vi "Add Transfer Group with Children v2.vi"(6 "Plugin Decimation (1)":u64=1, 7 "Transfer Group configuration":T1={"name"="", "direction"=enum."Tx", "cycle timing"={"priority"=0, "decimation"=1, "offset"=0}, "thread index"=-1, "settings"=[], "Transfers"=[], "timeout behavior"=enum."Increment Late Count"} {"Transfers"."channels"."string offset" format="%d bytes"}, 8 "error in (no error)":errorcluster, 9 "Transfer Group":refnum<class "Transfer Group.lvclass">, 10 "parent tag":string, 11 "Application Data In":T10) -> (0 "error out":errorcluster, 2 "average bandwidth":dbl format="%.0g bytes", 3 "Application Data In":T10)   [LabVIEW 2017, in "DSF Core.lvlib"]
uses:
  DSF Core.lvlib
  ID to Tree Items/Tree Item Type.ctl
  Classes/Transfer Group/Transfer Group.lvclass
  Classes/Timing/Timing.lvclass
  Classes/Buffers/Buffers.lvclass
  Buffer Reader/Buffer Data.ctl
  Classes/Transfer Group Status/Status.lvclass
  Classes/Buffer/Buffer.lvclass
  <vilib>/NI/Memory Manager/Classes/Pointer/Pointer.lvclass
  Main VI/Application Data.ctl
  Classes/Framework/Framework.lvclass
  Typedefs/DSF Timing Info.ctl
  Typedefs/DSF Settings Info.ctl
  Typedefs/DSF Engine Plugin Thread Configuration.ctl
  Typedefs/DSF Direction.ctl
  Typedefs/DSF Byte Order.ctl
  Typedefs/DSF Data Type.ctl
  Typedefs/DSF Engine Channel Configuration.ctl
  Typedefs/DSF Engine Transfer Configuration.ctl
  Typedefs/DSF Timeout Behavior.ctl
  Typedefs/DSF Engine Transfer Group Configuration.ctl
  Typedefs/DSF Engine Plugin Configuration.ctl
  Typedefs/DSF Engine Framework Configuration.ctl
panel:
  in  "plugin id":i32
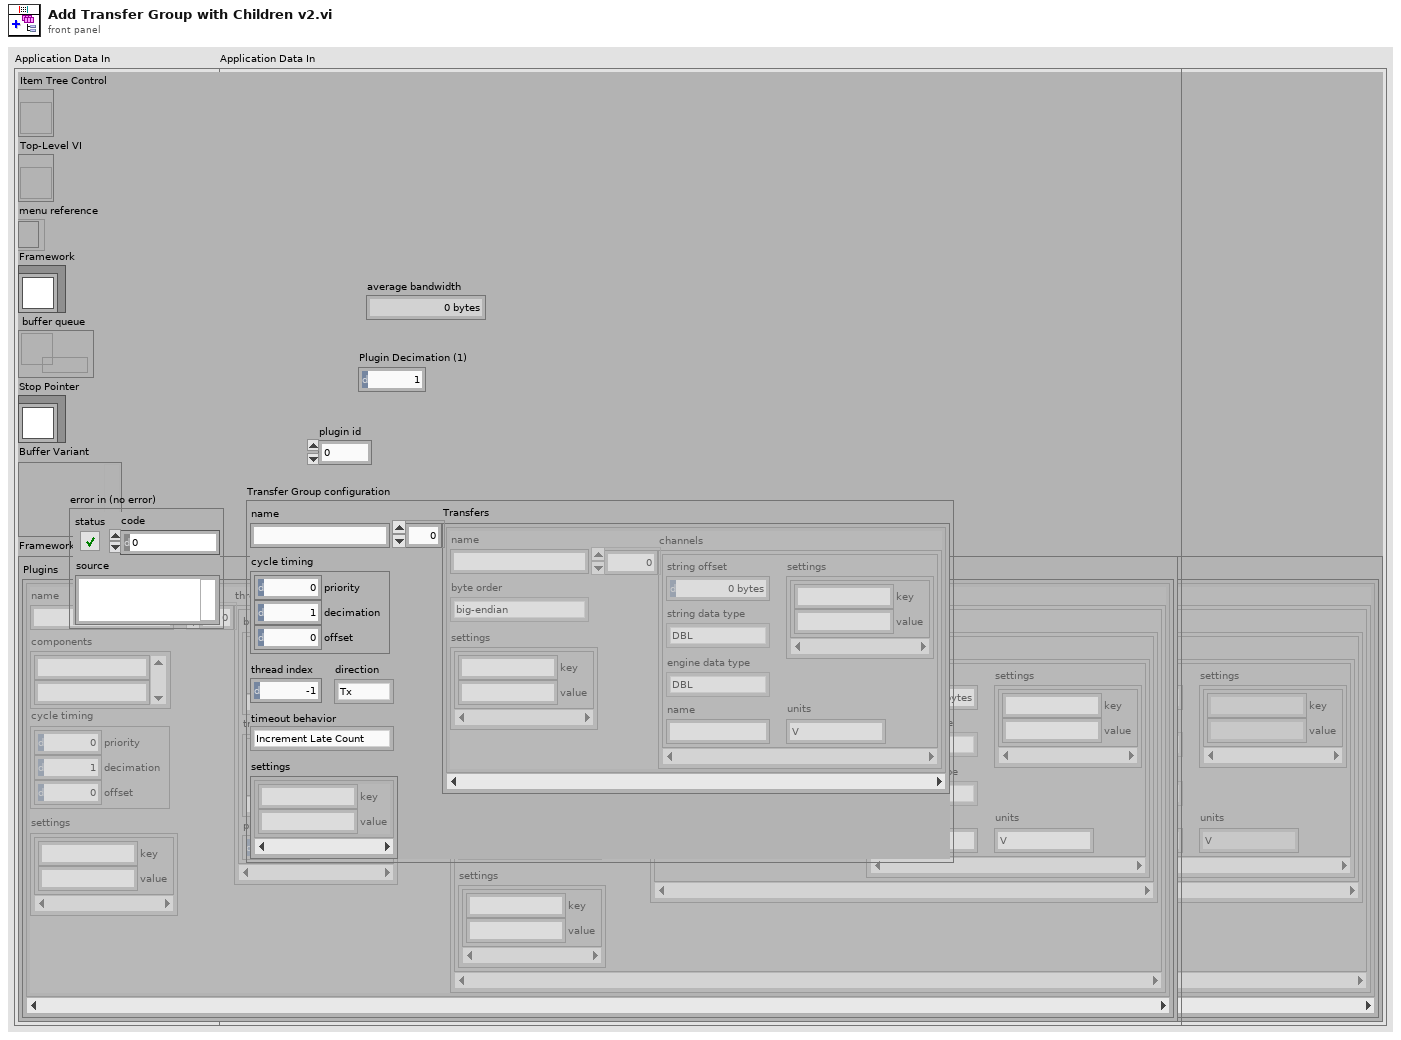
[diagram p1: front panel]
types:
  T1 = typedef "DSF Core.lvlib/DSF Engine Transfer Group Configuration.ctl" = cluster{"name":string, "direction":T2, "cycle timing":T3, "thread index":i32, "settings":T4, "Transfers":T5[], "timeout behavior":T9}
  T2 = typedef "DSF Core.lvlib/DSF Direction.ctl" = enum8{"Tx", "Rx"}
  T3 = typedef "DSF Core.lvlib/DSF Timing Info.ctl" = cluster{"priority":u64, "decimation":u64, "offset":u64}
  T4 = typedef "DSF Core.lvlib/DSF Settings Info.ctl" = cluster{"key":string, "value":string}[]
  T5 = typedef "DSF Core.lvlib/DSF Engine Transfer Configuration.ctl" = cluster{"name":string, "byte order":T6, "settings":T4, "channels":T7[]}
  T6 = typedef "DSF Core.lvlib/DSF Byte Order.ctl" = enum8{"big-endian", "little-endian"}
  T7 = typedef "DSF Core.lvlib/DSF Engine Channel Configuration.ctl" = cluster{"string offset":u64, "string data type":T8, "engine data type":T8, "name":string, "settings":T4, "units":string}
  T8 = typedef "DSF Core.lvlib/DSF Data Type.ctl" = enum8{"Bool", "SGL", "DBL", "I8", "I16", "I32", "I64", "U8", "U16", "U32", "U64"}
  T9 = typedef "DSF Core.lvlib/DSF Timeout Behavior.ctl" = enum8{"Increment Late Count", "Throw Error"}
  T10 = typedef "DSF Core.lvlib/Application Data.ctl" = cluster{"Item Tree Control":refnum<vi>, "Top-Level VI":refnum<vi>, "menu reference":refnum<k9>, "Framework":refnum<class "Framework.lvclass">, "buffer queue":refnum<queue>, "Stop Pointer":refnum<class "Pointer.lvclass">, "Buffer Variant":variant, "Framework Configuration":T11}
  T11 = typedef "DSF Core.lvlib/DSF Engine Framework Configuration.ctl" = cluster{"Plugins":T12[]}
  T12 = typedef "DSF Core.lvlib/DSF Engine Plugin Configuration.ctl" = cluster{"name":string, "components":string[], "cycle timing":T3, "threads":T13[], "Transfer Groups":T1[], "settings":T4}
  T13 = typedef "DSF Core.lvlib/DSF Engine Plugin Thread Configuration.ctl" = cluster{"buffer converter settings":T4, "transceiver settings":T4, "processor":i32, "priority offset":i16}
  T14 = typedef "DSF Core.lvlib/Buffer Data.ctl" = cluster{"Buffer":refnum<class "Buffer.lvclass">, "Status":refnum<class "Status.lvclass">, "decimation":u64, "avg bandwidth":dbl}
  T15 = typedef "DSF Core.lvlib/Tree Item Type.ctl" = enum16{"Framework", "Plugin Group", "Plugin", "Group", "Transfer", "Buffer", "Channel"}
  T16 = typedef "DSF Core.lvlib/Tree Item.ctl" = cluster{"Left Cell String":string, "Child Text":string[], "Child Tag":string, "Glyph Index":i32}
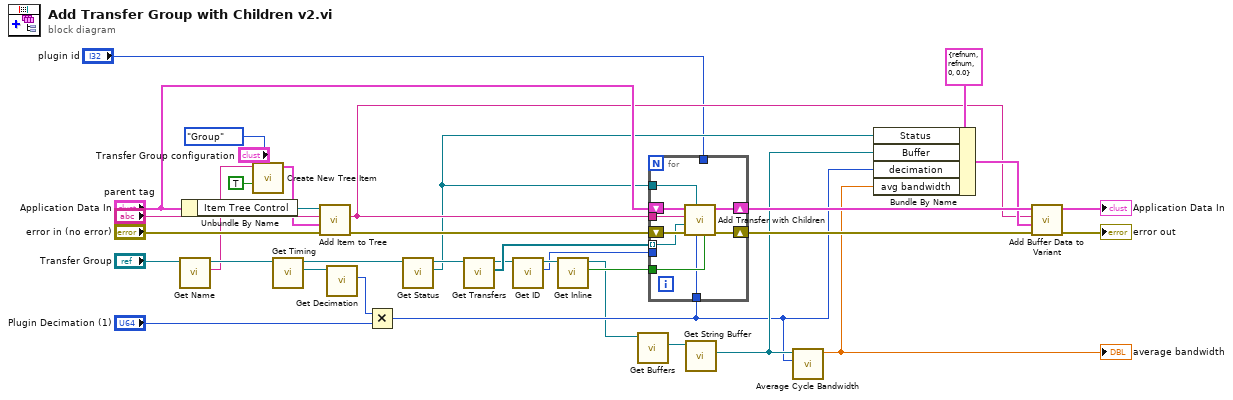
[diagram p0: block diagram]
diagram:
  n1 = call "Get Name.vi"("Transfer Group in"="Transfer Group") -> ("name"=w23:string, "Transfer Group out"=w26:refnum<class "Transfer Group.lvclass">)  [unwired: 9 in]
  n2 = Unbundle By Name("Application Data In") -> ("Item Tree Control"=w28:refnum<vi>)
  n3 = call "Create New Tree Item.vi"("Item Type"=Tree_Item_Type."Group", "found?"=TRUE, "Left Cell String"=w23) -> ("Item"=w30:T16)  [unwired: 7 in, 1 out]
  n4 = call "Get Timing.vi"("Transfer Group in"=w26) -> ("Timing"=w21:refnum<class "Timing.lvclass">, "Transfer Group out"=w14:refnum<class "Transfer Group.lvclass">)  [unwired: 9 in]
  n5 = call "Add Item to Tree.vi"("error in (no error)"="error in (no error)", "Item"=w30, "parent tag"="parent tag", "TreeControl in"=w28) -> ("error out"=w19:errorcluster, "new item tag"=w11:string)  [unwired: 5 in, 1 out]
  n6 = call "Get Decimation.vi"("Timing in"=w21) -> ("Decimation"=w25:u64)  [unwired: 9 in, 1 out]
  n7 = Multiply(x=w25, y="Plugin Decimation (1)") -> (x*y=w7:u64)
  n8 = call "Get Status.vi"("Transfer Group in"=w14) -> ("status pointer"=w10:refnum<class "Status.lvclass">, "Transfer Group out"=w13:refnum<class "Transfer Group.lvclass">)  [unwired: 9 in]
  n9 = call "Get Transfers.vi"("Transfer Group in"=w13) -> ("Transfers"=w29:refnum<class "Transfer.lvclass">[], "Transfer Group out"=w5:refnum<class "Transfer Group.lvclass">)  [unwired: 9 in]
  n10 = call "Get ID.vi"("Transfer Group in"=w5) -> ("id"=w2:i32, "Transfer Group out"=w3:refnum<class "Transfer Group.lvclass">)  [unwired: 9 in]
  n11 = call "Get Inline.vi"("Transfer Group in"=w3) -> ("inline"=w6:bool, "Transfer Group out"=w4:refnum<class "Transfer Group.lvclass">)  [unwired: 9 in]
  n12 = call "Get Buffers.vi"("Transfer Group in"=w4) -> ("Buffers"=w22:refnum<class "Buffers.lvclass">)  [unwired: 9 in, 1 out]
  n13 = for {
    shift-right: [w42] -> w18
    shift-left: "Application Data In" -> [w44]
    shift-right: [w41] -> w17
    shift-left: w19 -> [w43]
    tunnel: w29 -> [w40] mode=indexing
    tunnel: w11 -> [w39]
    tunnel: w6 -> [w38]
    tunnel: w7 -> [w37]
    tunnel: w10 -> [w36]
    tunnel: w2 -> [_]
    tunnel: "plugin id" -> [_]
    n14 = call "Add Transfer with Children.vi"("inline"=w38, "Group Decimation (1)"=w37, "Transfer Group Status"=w36, "error in (no error)"=w43, "Transfer"=w40, "parent tag"=w39, "Application Data In"=w44) -> ("error out"=w41:errorcluster, "Application Data Out"=w42:T10)  [unwired: 3 in]
  }
  n15 = call "Get String Buffer.vi"("Buffers in"=w22) -> ("String Buffer"=w8:refnum<class "Buffer.lvclass">)  [unwired: 9 in, 1 out]
  n16 = call "Average Cycle Bandwidth.vi"("Decimation"=w7, "Buffer"=w8) -> ("avergage cycle bandwidth"=w9:dbl)  [unwired: 9 in]
  "average bandwidth" <- w9
  n17 = Bundle By Name(cluster=T14 {"Buffer"=refnum, "Status"=refnum, "decimation"=0, "avg bandwidth"=0.0} ("Buffer data"), "Status"=w10, "Buffer"=w8, "decimation"=w7, "avg bandwidth"=w9) -> (w12:T14)
  n18 = call "Add Buffer Data to Variant.vi"("error in (no error)"=w17, "Buffer data"=w12, "tag"=w11, "Application Data In in"=w18) -> ("error out"=→"error out":errorcluster, "Application Data In out"=→"Application Data In":T10)  [unwired: 6 in]
